vi "Main.vi"(8 "error":errorcluster) -> (0 "Error out":errorcluster)   [LabVIEW 2018, in "S1.lvclass"]
doc: "Use this template to build a simple state machine design pattern. Each state executes code and determines which state to transition to."
uses:
  S1.lvclass
  S1.lvclass/S1.ctl
  Controller/Public Controls/S1Config.ctl
  Controller/Public Controls/GlobalConfig.ctl
  Public Controls/Outputs.ctl
  Public Controls/ReportHeader.ctl
  Controller/Public Controls/TestInfo.ctl
  ce2ffe4b-55ea-4b97-aeef-069ef36f3054.vi
  18d9e863-2333-4af4-97b0-9e95cfa094dc.vi
  <vilib>/Utility/file.llb/Write Delimited Spreadsheet (string).vi
  Controller/GUI.lvclass
  IO/IO.lvclass
panel:
  out "Loop":i32
  # "S1 MAIN"
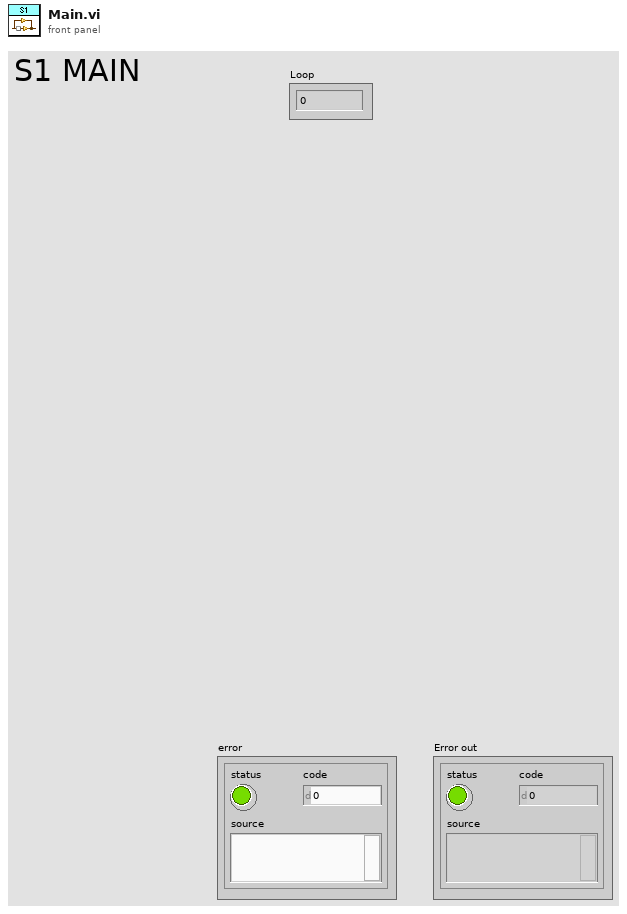
[diagram p1: front panel]
types:
  T1 = typedef "S1.lvclass/Outputs.ctl" = cluster{"LoP":bool, "HiP":bool, "Z1Vent":bool, "Z2Vent":bool, "Z3Vent":bool, "IsLidLock":bool}
  T2 = typedef "S1.lvclass/ReportHeader.ctl" = string
  T3 = typedef "GUI.lvclass/TestInfo.ctl" = cluster{"TestType":string, "SN":string}
  T4 = typedef "S1.lvclass/State.ctl" = enum16{"Initialize", "SetConfig", "AckAlarm", "Alarm", "Idle", "LockLid", "LowPressure", "HighPressure", "Vent", "Abort", "Start", "CreateReports", "WriteToReport", "WritePressure", "Error", "Exit"}
  T5 = typedef "GUI.lvclass/GlobalConfig.ctl" = cluster{"Report Folder Path":path, "PT1_MIN":dbl, "PT1_MAX":dbl, "VENT_PMAX":dbl, "LOP_TARGET":dbl, "LOP_RAMP":dbl, "LOP_LEAK_MAX":dbl, "HIP_TARGET":dbl, "HIP_RAMP":dbl, "HIP_MIN":dbl, "HIP_MAX":dbl, "BLEED_TIME":dbl, "LOP_MAX":dbl, "LOP_MIN":dbl, "PT131Com":refnum<visa-resource-name>, "PT231Com":refnum<visa-resource-name>, "PT331Com":refnum<visa-resource-name>, "PT431Com":refnum<visa-resource-name>, "PT531Com":refnum<visa-resource-name>, "PT631Com":refnum<visa-resource-name>}
  T6 = typedef "GUI.lvclass/S1Config.ctl" = cluster{"S1Z3_VENT_PMAX":dbl, "MSLOP_TIMER":dbl, "S1Z3_LOP_LEAK_MAX":dbl, "MSHIP_TIMER":dbl, "TJLOP_TIMER":dbl, "TJHIP_TIMER":dbl, "TJ_PTEST_MAX":dbl, "TJHIP_STABLE_WAIT":dbl, "TJHIP_STABLE_CLOSE":dbl}
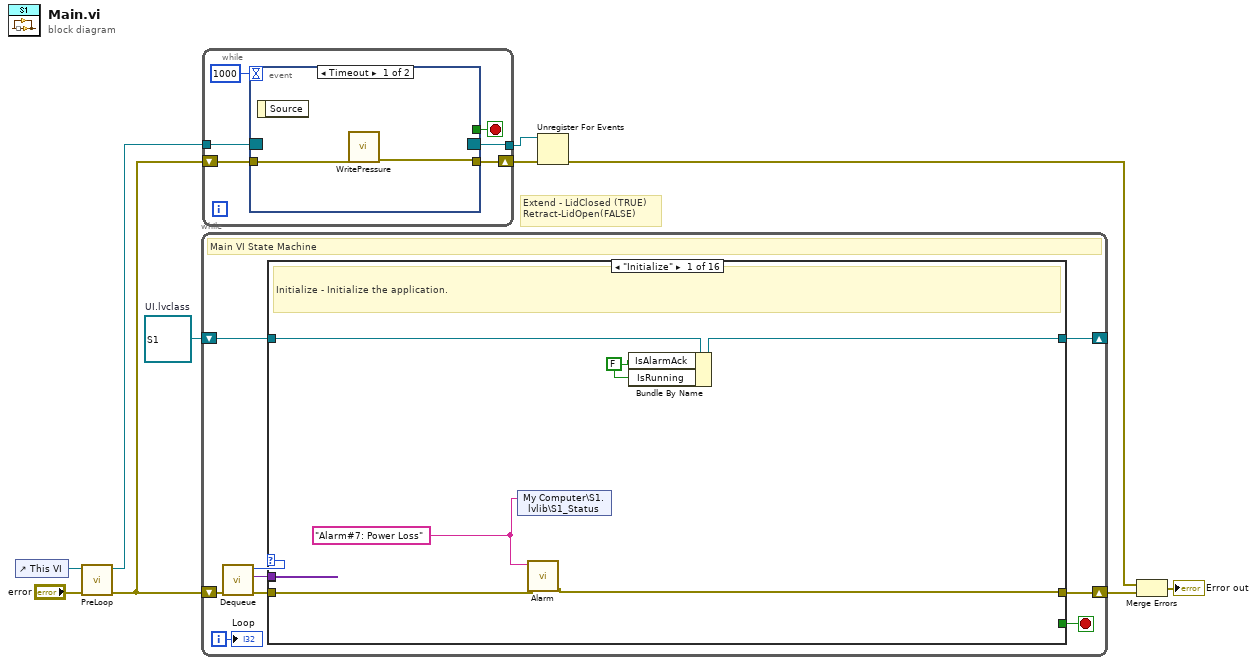
[diagram p0: block diagram]
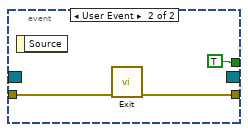
[diagram p2: hidden frame]
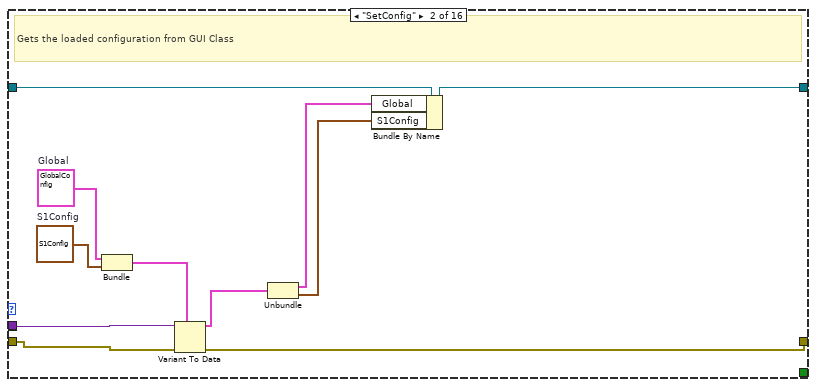
[diagram p3: hidden frame]
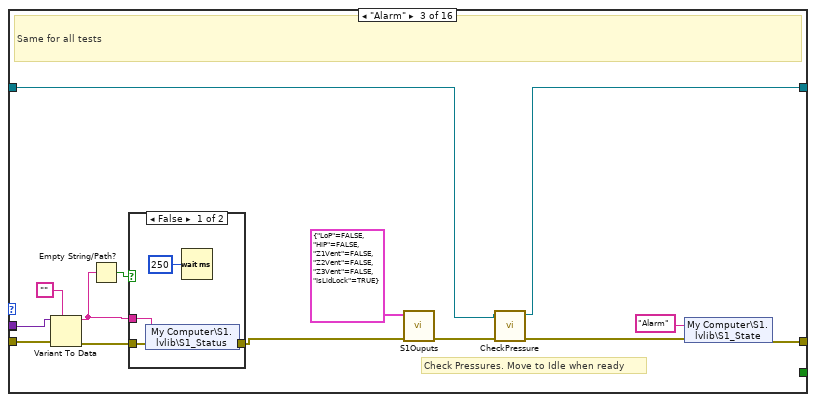
[diagram p4: hidden frame]
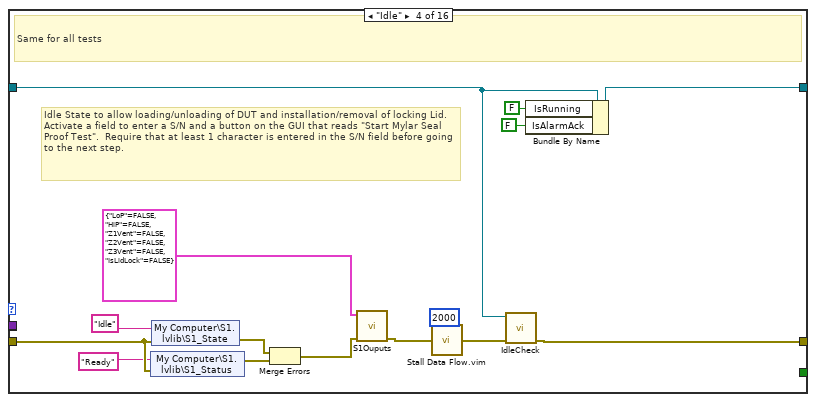
[diagram p6: hidden frame]
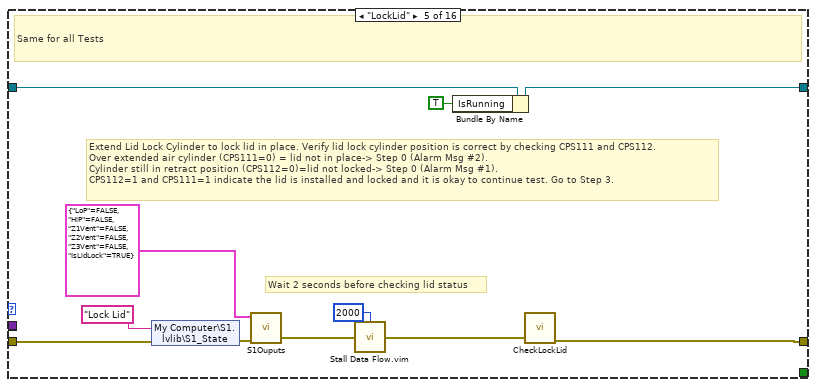
[diagram p7: hidden frame]
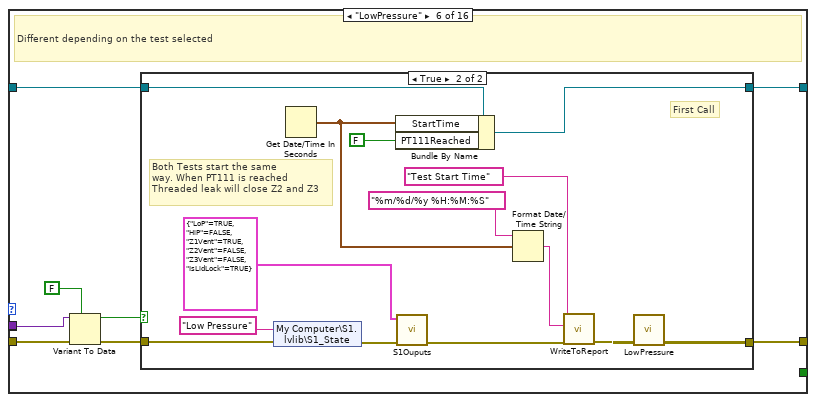
[diagram p8: hidden frame]
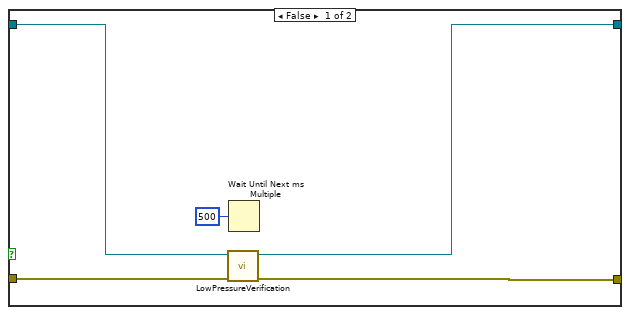
[diagram p9: hidden frame]
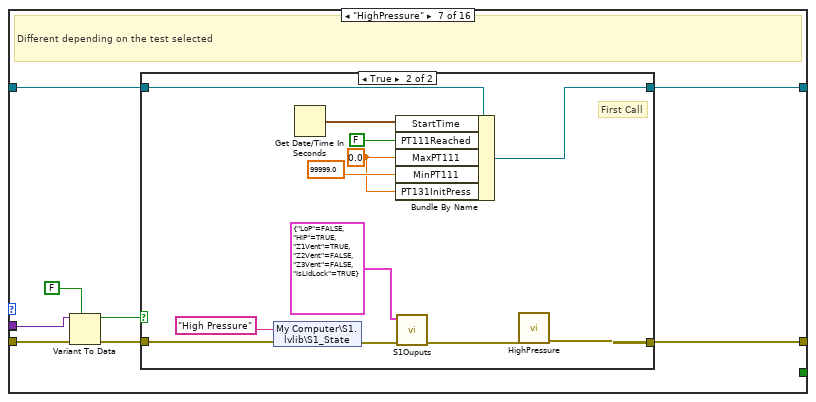
[diagram p10: hidden frame]
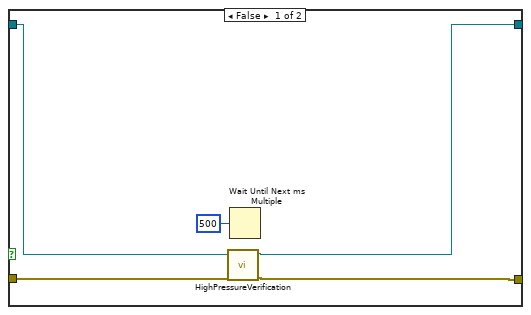
[diagram p11: hidden frame]
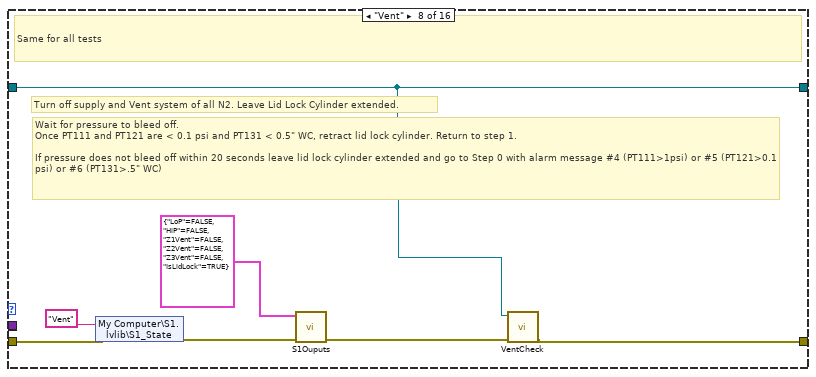
[diagram p12: hidden frame]
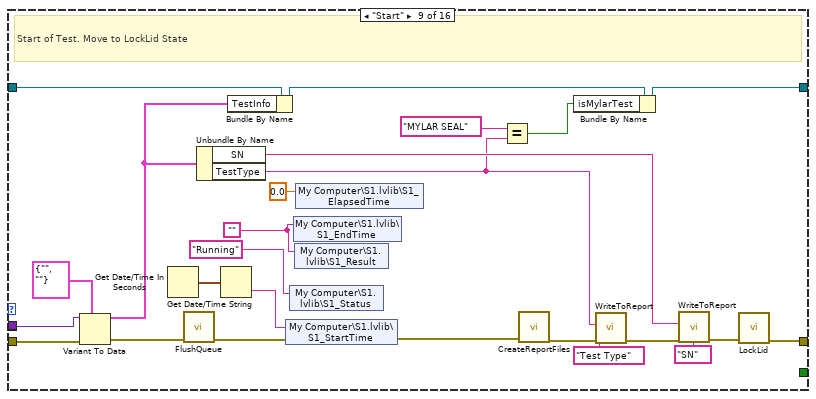
[diagram p13: hidden frame]
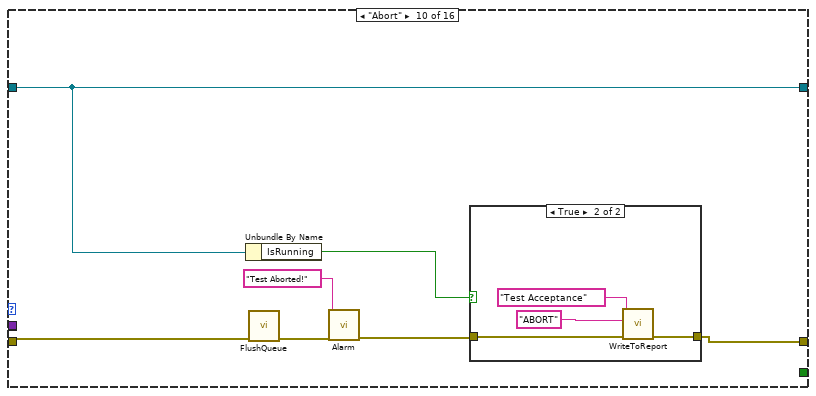
[diagram p14: hidden frame]
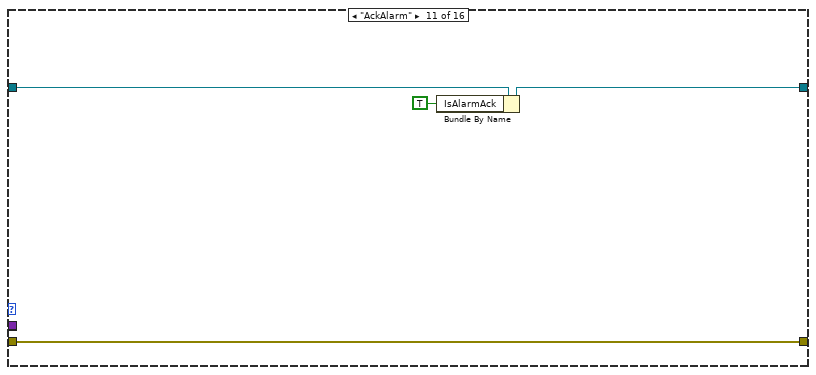
[diagram p16: hidden frame]
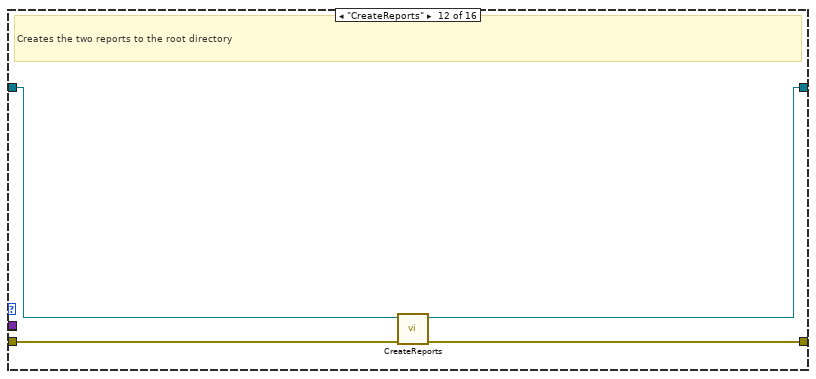
[diagram p17: hidden frame]
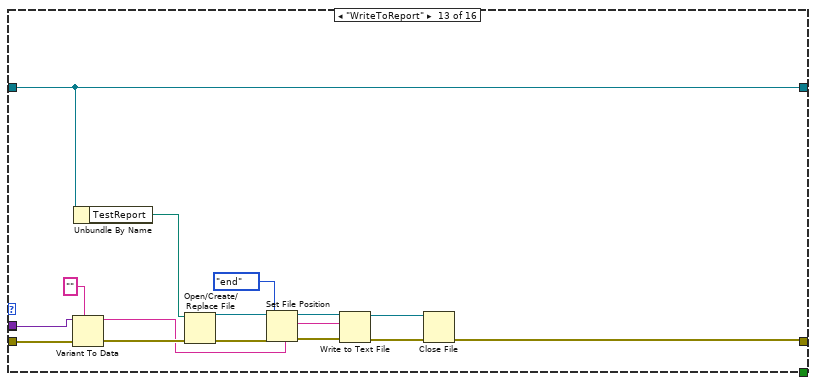
[diagram p18: hidden frame]
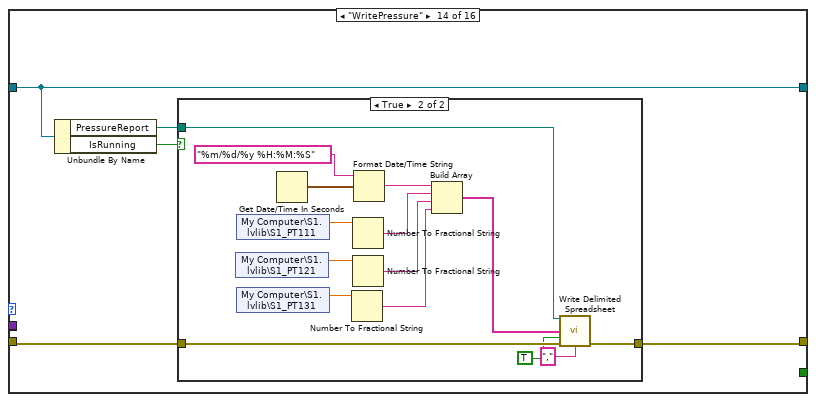
[diagram p19: hidden frame]
diagram:
  w10 = refnum<class "S1.lvclass"> refnum  # UI.lvclass
  # "Extend - LidClosed (TRUE)\nRetract-LidOpen(FALSE)"
  n1 = control-ref of="This VI"() -> (w7:refnum<vi>)
  n2 = call "PreLoop.vi"("error in"="error", "VI Ref"=w7) -> ("error out"=w6:errorcluster, "Event Registration Refnum"=w8:refnum<event-registration>)  [unwired: 8 in]
  n3 = while {
    shift-right: [w19] -> w3
    shift-left: w6 -> [w15]
    shift-right: [w16] -> _
    shift-left: w10 -> [w17]
    i -> [w11]
    stop <- w18 stop-if-true
    # "Main VI State Machine"
    n4 = call "Dequeue.vi"("error in"=w15) -> ("error out"=w14:errorcluster, "Data"=w12:variant, "State"=w13:T4)  [unwired: 8 in]
    n5 = case shown="\"Initialize\"" w13 {
      tunnel: [_ _ _ _ _ _ _ _ _ _ _ _ _ _ w224 _] -> w18
      tunnel: w14 -> [w23 w35 w43 w68 w80 w88 w115 w140 w161 w166 w181 w184 w198 w204 w222 w230]
      tunnel: [w22 w26 w44 w60 w76 w89 w116 w136 w150 w170 w181 w183 w191 w203 w222 w226] -> w19
      tunnel: w17 -> [w25 w36 w47 w56 w81 w83 w110 w134 w165 w169 w180 w185 w197 w205 w223 w233]
      tunnel: [w24 w30 w46 w63 w73 w82 w109 w134 w144 w169 w179 w182 w197 w205 w223 w233] -> w16
      tunnel: w12 -> [_ w34 w42 _ _ w87 w114 _ w159 _ _ _ w199 _ _ w229]
      tunnel: w12 -> [_ _ _ _ _ _ _ _ _ _ _ _ _ _ _ _]
      frame "Initialize" {
        w20 = FALSE ("IsAlarmAck")
        w21 = "Alarm#7: Power Loss" ("Status")
        # "Initialize - Initialize the application."
        n6 = shared-variable "My Computer\\S1.lvlib\\S1_Status"(w21) -> ()  [unwired: 1 in, 1 out]
        n7 = call "Alarm.vi"("error in"=w23, "Alarm"=w21) -> ("error out"=w22:errorcluster)  [unwired: 9 in]
        n8 = Bundle By Name(cluster=w25, "IsAlarmAck"=w20, "IsRunning"=w20) -> (w24:refnum<class "S1.lvclass">)
      }
      frame "SetConfig" {
        w33 = T5 {"Report Folder Path"=path "", "PT1_MIN"=0.0, "PT1_MAX"=0.0, "VENT_PMAX"=0.0, "LOP_TARGET"=0.0, "LOP_RAMP"=0.0, "LOP_LEAK_MAX"=0.0, "HIP_TARGET"=0.0, "HIP_RAMP"=0.0, "HIP_MIN"=0.0, "HIP_MAX"=0.0, "BLEED_TIME"=0.0, "LOP_MAX"=0.0, "LOP_MIN"=0.0, "PT131Com"="COM5", "PT231Com"="COM6", "PT331Com"="COM7", "PT431Com"="COM8", "PT531Com"="COM9", "PT631Com"="COM10"}  # Global
        w32 = T6 {"S1Z3_VENT_PMAX"=0.0, "MSLOP_TIMER"=0.0, "S1Z3_LOP_LEAK_MAX"=0.0, "MSHIP_TIMER"=0.0, "TJLOP_TIMER"=0.0, "TJHIP_TIMER"=0.0, "TJ_PTEST_MAX"=0.0, "TJHIP_STABLE_WAIT"=0.0, "TJHIP_STABLE_CLOSE"=0.0}  # S1Config
        # "Gets the loaded configuration from GUI Class"
        n9 = Bundle("Global"=w33, "S1Config"=w32) -> (w31:cluster{"Global":T5, "S1Config":T6})  [unwired: 1 in]
        n10 = Variant To Data(error in=w35, type=w31, Variant=w34) -> (data=w29:cluster{"Global":T5, "S1Config":T6}, error out=w26:errorcluster)
        n11 = Unbundle(w29) -> ("Global"=w28:T5, "S1Config"=w27:T6)
        n12 = Bundle By Name(cluster=w36, "Global"=w28, "S1Config"=w27) -> (w30:refnum<class "S1.lvclass">)
      }
      frame "Alarm" {
        # "Check Pressures. Move to Idle when ready"
        # "Same for all tests"
        n13 = Variant To Data(error in=w43, type="", Variant=w42) -> (data=w39:string, error out=w38:errorcluster)
        n14 = Empty String/Path?(string/path=w39) -> (empty?=w40:bool)
        n15 = case shown="False" w40 {
          tunnel: w39 -> [w54 _]
          tunnel: w38 -> [w53 w55]
          tunnel: [w52 w55] -> w37
          frame False {
            n16 = shared-variable "My Computer\\S1.lvlib\\S1_Status"(w54, error in=w53) -> (error out=w52:errorcluster)
            n17 = Wait (ms)(milliseconds to wait=u32 250) -> ()  [unwired: 1 out]
          }
          frame True {
          }
        }
        n18 = call "S1Ouputs.vi"("error in"=w37, "SIOutputs"=T1 {"LoP"=FALSE, "HiP"=FALSE, "Z1Vent"=FALSE, "Z2Vent"=FALSE, "Z3Vent"=FALSE, "IsLidLock"=TRUE}) -> ("error out"=w48:errorcluster)  [unwired: 9 in]
        n19 = call "CheckPressure.vi"("error in (no error)"=w48, "UI.lvclass"=w47) -> ("error out"=w45:errorcluster, "UI.lvclass"=w46:refnum<class "S1.lvclass">)  [unwired: 8 in]
        n20 = shared-variable "My Computer\\S1.lvlib\\S1_State"("Alarm" ("S1Status"), error in=w45) -> (error out=w44:errorcluster)
      }
      frame "Idle" {
        # "Idle State to allow loading/unloading of DUT and installation/removal of locking Lid.  Activate a field to enter a S/N and a button on the GUI that reads \"Start Mylar Seal Proof Test\".  Require that at least 1 character is entered in the S/N field before going to the next step."
        # "Same for all tests"
        n21 = shared-variable "My Computer\\S1.lvlib\\S1_Status"("Ready" ("Status"), error in=w68) -> (error out=w66:errorcluster)
        n22 = shared-variable "My Computer\\S1.lvlib\\S1_State"("Idle" ("S1Status"), error in=w68) -> (error out=w67:errorcluster)
        n23 = Merge Errors(w67, w66) -> (w65:errorcluster)
        n24 = call "S1Ouputs.vi"("error in"=w65, "SIOutputs"=T1 {"LoP"=FALSE, "HiP"=FALSE, "Z1Vent"=FALSE, "Z2Vent"=FALSE, "Z3Vent"=FALSE, "IsLidLock"=FALSE}) -> ("error out"=w61:errorcluster)  [unwired: 9 in]
        n25 = call "Stall Data Flow.vim"("value in"=w61, "milliseconds to wait"=u32 2000) -> ("value out"=w58:errorcluster)  [unwired: 1 out]
        n26 = call "IdleCheck.vi"("error in (no error)"=w58, "S1.lvclass"=w56) -> ("error out"=w60:errorcluster)  [unwired: 9 in]
        n27 = Bundle By Name(cluster=w56, "IsRunning"=FALSE, "IsAlarmAck"=FALSE) -> (w63:refnum<class "S1.lvclass">)
      }
      frame "LockLid" {
        # "Wait 2 seconds before checking lid status"
        # "Extend Lid Lock Cylinder to lock lid in place. Verify lid lock cylinder position is correct by checking CPS111 and CPS112. \nOver extended air cylinder (CPS111=0) = lid not in place-> Step 0 (Alarm Msg #2). \nCylinder still in retract position (CPS112=0)=lid not locked-> Step 0 (Alarm Msg #1). \nCPS112=1 and CPS111=1 indicate the lid is installed and locked and it is okay to continue test. Go to Step 3."
        # "Same for all Tests"
        n28 = shared-variable "My Computer\\S1.lvlib\\S1_State"("Lock Lid" ("S1Status"), error in=w80) -> (error out=w78:errorcluster)
        n29 = call "S1Ouputs.vi"("error in"=w78, "SIOutputs"=T1 {"LoP"=FALSE, "HiP"=FALSE, "Z1Vent"=FALSE, "Z2Vent"=FALSE, "Z3Vent"=FALSE, "IsLidLock"=TRUE}) -> ("error out"=w75:errorcluster)  [unwired: 9 in]
        n30 = call "Stall Data Flow.vim"("value in"=w75, "milliseconds to wait"=u32 2000) -> ("value out"=w74:errorcluster)  [unwired: 1 out]
        n31 = Bundle By Name(cluster=w81, "IsRunning"=TRUE) -> (w73:refnum<class "S1.lvclass">)
        n32 = call "CheckLockLid.vi"("error in (no error)"=w74) -> ("error out"=w76:errorcluster)  [unwired: 10 in]
      }
      frame "LowPressure" {
        # "Different depending on the test selected"
        n33 = Variant To Data(error in=w88, type=FALSE, Variant=w87) -> (data=w84:bool, error out=w85:errorcluster)
        n34 = case shown="True" w84 {
          tunnel: [w93 w95] -> w89
          tunnel: w85 -> [w94 w106]
          tunnel: w83 -> [w92 w99]
          tunnel: [w91 w105] -> w82
          frame False {
            n35 = call "LowPressureVerification.vi"("error in"=w94, "S1 in"=w92) -> ("error out"=w93:errorcluster, "S1 out"=w91:refnum<class "S1.lvclass">)  [unwired: 8 in]
            n36 = Wait Until Next ms Multiple(millisecond multiple=u32 500) -> ()  [unwired: 1 out]
          }
          frame True {
            # "Both Tests start the same\nway. When PT111 is reached\nThreaded leak will close Z2 and Z3"
            # "First Call"
            n37 = shared-variable "My Computer\\S1.lvlib\\S1_State"("Low Pressure" ("S1Status"), error in=w106) -> (error out=w107:errorcluster)
            n38 = Get Date/Time In Seconds() -> (seconds since 1Jan1904=w102:timestamp)
            n39 = Bundle By Name(cluster=w99, "StartTime"=w102, "PT111Reached"=FALSE ("PT111ReachedPressure")) -> (w105:refnum<class "S1.lvclass">)
            n40 = call "S1Ouputs.vi"("error in"=w107, "SIOutputs"=T1 {"LoP"=TRUE, "HiP"=FALSE, "Z1Vent"=TRUE, "Z2Vent"=FALSE, "Z3Vent"=FALSE, "IsLidLock"=TRUE}) -> ("error out"=w97:errorcluster)  [unwired: 9 in]
            n41 = Format Date/Time String(time format string (%c)="%m/%d/%y %H:%M:%S", seconds (now)=w102) -> (date/time string=w101:string)  [unwired: 1 in]
            n42 = call "WriteToReport.vi"("error in"=w97, "Value"=w101, "Header"=T2 "Test Start Time") -> ("error out"=w96:errorcluster)  [unwired: 8 in]
            n43 = call "LowPressure.vi"("error in"=w96) -> ("error out"=w95:errorcluster)  [unwired: 10 in]
          }
        }
      }
      frame "HighPressure" {
        # "Different depending on the test selected"
        n44 = Variant To Data(error in=w115, type=FALSE, Variant=w114) -> (data=w111:bool, error out=w112:errorcluster)
        n45 = case shown="True" w111 {
          tunnel: [w118 w125] -> w116
          tunnel: w112 -> [w119 w131]
          tunnel: w110 -> [w121 w124]
          tunnel: [w120 w130] -> w109
          frame False {
            n46 = call "HighPressureVerification.vi"("error in"=w119, "S1 in"=w121) -> ("error out"=w118:errorcluster, "S1 out"=w120:refnum<class "S1.lvclass">)  [unwired: 8 in]
            n47 = Wait Until Next ms Multiple(millisecond multiple=u32 500) -> ()  [unwired: 1 out]
          }
          frame True {
            w122 = 0.0 ("MaxPT111")
            # "First Call"
            n48 = shared-variable "My Computer\\S1.lvlib\\S1_State"("High Pressure" ("S1Status"), error in=w131) -> (error out=w132:errorcluster)
            n49 = Get Date/Time In Seconds() -> (seconds since 1Jan1904=w129:timestamp)
            n50 = Bundle By Name(cluster=w124, "StartTime"=w129, "PT111Reached"=FALSE ("PT111ReachedPressure"), "MaxPT111"=w122, "MinPT111"=99999.0, "PT131InitPress"=w122) -> (w130:refnum<class "S1.lvclass">)
            n51 = call "S1Ouputs.vi"("error in"=w132, "SIOutputs"=T1 {"LoP"=FALSE, "HiP"=TRUE, "Z1Vent"=TRUE, "Z2Vent"=FALSE, "Z3Vent"=FALSE, "IsLidLock"=TRUE}) -> ("error out"=w128:errorcluster)  [unwired: 9 in]
            n52 = call "HighPressure.vi"("error in"=w128) -> ("error out"=w125:errorcluster)  [unwired: 10 in]
          }
        }
      }
      frame "Vent" {
        # "Wait for pressure to bleed off. \nOnce PT111 and PT121 are < 0.1 psi and PT131 < 0.5\" WC, retract lid lock cylinder. Return to step 1. \n\nIf pressure does not bleed off within 20 seconds leave lid lock cylinder extended and go to Step 0 with alarm message #4 (PT111>1psi) or #5 (PT121>0.1 psi) or #6 (PT131>.5\" WC)"
        # "Turn off supply and Vent system of all N2. Leave Lid Lock Cylinder extended."
        # "Same for all tests"
        n53 = shared-variable "My Computer\\S1.lvlib\\S1_State"("Vent" ("S1Status"), error in=w140) -> (error out=w138:errorcluster)
        n54 = call "S1Ouputs.vi"("error in"=w138, "SIOutputs"=T1 {"LoP"=FALSE, "HiP"=FALSE, "Z1Vent"=FALSE, "Z2Vent"=FALSE, "Z3Vent"=FALSE, "IsLidLock"=TRUE}) -> ("error out"=w135:errorcluster)  [unwired: 9 in]
        n55 = call "VentCheck.vi"("error in (no error)"=w135, "UI.lvclass"=w134) -> ("error out"=w136:errorcluster)  [unwired: 9 in]
      }
      frame "Start" {
        w147 = ""
        # "Start of Test. Move to LockLid State"
        n56 = Variant To Data(error in=w161, type=T3 {"TestType"="", "SN"=""} ("TestInfo"), Variant=w159) -> (data=w155:T3, error out=w142:errorcluster)
        n57 = Get Date/Time In Seconds() -> (seconds since 1Jan1904=w164:timestamp)
        n58 = call "FlushQueue.vi"("error in"=w142) -> ("error out"=w141:errorcluster)  [unwired: 10 in]
        n59 = Unbundle By Name(w155) -> ("SN"=w153:string, "TestType"=w145:string)
        n60 = Get Date/Time String(seconds (now)=w164) -> (time string=w163:string)  [unwired: 2 in, 1 out]
        n61 = Bundle By Name(cluster=w165, "TestInfo"=w155) -> (w158:refnum<class "S1.lvclass">)
        n62 = shared-variable "My Computer\\S1.lvlib\\S1_StartTime"(w163, error in=w141) -> (error out=w149:errorcluster)
        n63 = shared-variable "My Computer\\S1.lvlib\\S1_Status"("Running" ("S1Status")) -> ()  [unwired: 1 in, 1 out]
        n64 = shared-variable "My Computer\\S1.lvlib\\S1_EndTime"(w147) -> ()  [unwired: 1 in, 1 out]
        n65 = shared-variable "My Computer\\S1.lvlib\\S1_Result"(w147) -> ()  [unwired: 1 in, 1 out]
        n66 = shared-variable "My Computer\\S1.lvlib\\S1_ElapsedTime"(0.0 ("ElapsedTime")) -> ()  [unwired: 1 in, 1 out]
        n67 = Equal?(x="MYLAR SEAL" ("TestInfo.TestType"), y=w145) -> (x = y?=w143:bool)
        n68 = call "CreateReportFiles.vi"("error in"=w149) -> ("error out"=w156:errorcluster)  [unwired: 10 in]
        n69 = Bundle By Name(cluster=w158, "isMylarTest"=w143) -> (w144:refnum<class "S1.lvclass">)
        n70 = call "WriteToReport.vi"("error in"=w156, "Value"=w145, "Header"="Test Type") -> ("error out"=w154:errorcluster)  [unwired: 8 in]
        n71 = call "WriteToReport.vi"("error in"=w154, "Value"=w153, "Header"="SN") -> ("error out"=w151:errorcluster)  [unwired: 8 in]
        n72 = call "LockLid.vi"("error in"=w151) -> ("error out"=w150:errorcluster)  [unwired: 10 in]
      }
      frame "Abort" {
        n73 = Unbundle By Name(w169) -> ("IsRunning"=w172:bool)
        n74 = call "FlushQueue.vi"("error in"=w166) -> ("error out"=w168:errorcluster)  [unwired: 10 in]
        n75 = call "Alarm.vi"("error in"=w168, "Alarm"="Test Aborted!" ("S1Status")) -> ("error out"=w171:errorcluster)  [unwired: 9 in]
        n76 = case shown="True" w172 {
          tunnel: w171 -> [w173 w177]
          tunnel: [w173 w176] -> w170
          frame False {
          }
          frame True {
            n77 = call "WriteToReport.vi"("error in"=w177, "Value"="ABORT", "Header"=T2 "Test Acceptance") -> ("error out"=w176:errorcluster)  [unwired: 8 in]
          }
        }
      }
      frame "AckAlarm" {
        n78 = Bundle By Name(cluster=w180, "IsAlarmAck"=TRUE) -> (w179:refnum<class "S1.lvclass">)
      }
      frame "CreateReports" {
        # "Creates the two reports to the root directory"
        n79 = call "CreateReports.vi"("error in (no error)"=w184, "S1 in"=w185) -> ("error out"=w183:errorcluster, "S1 out"=w182:refnum<class "S1.lvclass">)  [unwired: 8 in]
      }
      frame "WriteToReport" {
        n80 = Variant To Data(error in=w198, type="", Variant=w199) -> (data=w194:string, error out=w195:errorcluster)
        n81 = Unbundle By Name(w197) -> ("TestReport"=w196:path)
        n82 = Open/Create/Replace File(file path (use dialog)=w196, error in=w195) -> (refnum out=w187:refnum<file>, error out=w190:errorcluster)  [unwired: 4 in, 1 out]
        n83 = Set File Position(refnum=w187, from (0:start)=enum16{"start", "end", "current"}."end", error in=w190) -> (refnum out=w186:refnum<file>, error out=w188:errorcluster)  [unwired: 1 in]
        n84 = Write to Text File(file (use dialog)=w186, text=w194, error in=w188) -> (refnum out=w193:refnum<file>, error out=w192:errorcluster)  [unwired: 1 in, 1 out]
        n85 = Close File(refnum=w193, error in=w192) -> (error out=w191:errorcluster)  [unwired: 1 out]
      }
      frame "WritePressure" {
        n86 = Unbundle By Name(w205) -> ("PressureReport"=w201:path, "IsRunning"=w202:bool)
        n87 = case shown="True" w202 {
          tunnel: w204 -> [w206 w211]
          tunnel: [w206 w210] -> w203
          tunnel: w201 -> [_ w207]
          frame False {
          }
          frame True {
            n88 = shared-variable "My Computer\\S1.lvlib\\S1_PT121"() -> (w218:dbl)  [unwired: 1 in, 1 out]
            n89 = shared-variable "My Computer\\S1.lvlib\\S1_PT111"() -> (w219:dbl)  [unwired: 1 in, 1 out]
            n90 = shared-variable "My Computer\\S1.lvlib\\S1_PT131"() -> (w217:dbl)  [unwired: 1 in, 1 out]
            n91 = Get Date/Time In Seconds() -> (seconds since 1Jan1904=w221:timestamp)
            n92 = Number To Fractional String(number=w217) -> (F-format string=w213:string)  [unwired: 3 in]
            n93 = Number To Fractional String(number=w219) -> (F-format string=w215:string)  [unwired: 3 in]
            n94 = Number To Fractional String(number=w218) -> (F-format string=w214:string)  [unwired: 3 in]
            n95 = Format Date/Time String(time format string (%c)="%m/%d/%y %H:%M:%S", seconds (now)=w221) -> (date/time string=w216:string)  [unwired: 1 in]
            n96 = Build Array(w216, w215, w214, w213) -> (w212:string[])
            n97 = call-poly <vilib>:"Write Delimited Spreadsheet.vi"("file path (dialog if empty)"=w207, "1D data"=w212, "append to file? (new file:F)"=TRUE, "error in (no error)"=w211, "delimiter (\\t)"="," ("delimiter (\\t)")) -> ("error out"=w210:errorcluster)  [unwired: 9 in, 1 out]
          }
        }
      }
      frame "Exit" {
        w224 = TRUE  # Stop Loop
        # "Exit - Exit the application.\nSave / Close any files"
      }
      frame "Error" {
        n98 = Variant To Data(error in=w230, type=errorcluster {"status"=FALSE, "code"=0, "source"=""} ("error out"), Variant=w229) -> (data=w231:errorcluster, error out=w227:errorcluster)
        n99 = Unbundle By Name(w231) -> ("code"=w225:i32, "source"=w228:string)
        n100 = case shown="Default" w225 {
          tunnel: w228 -> [_ w235]
          tunnel: w227 -> [w234 w238]
          tunnel: [w234 w238] -> w226
          frame 1 {
            # "Error talking to other modules. \n\nIgnore. If testing by itself."
          }
          frame Default {
            n101 = Concatenate Strings("Error On Station 1 ", w235) -> (w237:string)
            n102 = One Button Dialog(message=w237) -> ()  [unwired: 1 in, 1 out]
          }
        }
      }
    }
    "Loop" <- w11
  }
  n103 = while {
    tunnel: w8 -> [w240]
    shift-right: [w242] -> w5
    shift-left: w6 -> [w244]
    tunnel: [w241] -> w4
    stop <- w243 stop-if-true
    n104 = event shown="[0] Timeout" {
      selector: w240 -> [_ _]
      dyn-events: [_ _] -> w241
      timeout: 1000 -> [_ _]
      tunnel: w244 -> [w246 w249]
      tunnel: [w245 w248] -> w242
      tunnel: [_ TRUE] -> w243
      event Timeout {
        n105 = event-data() -> ()  [unwired: 1 in, 1 out]
        n106 = call "WritePressure.vi"("error in"=w246) -> ("error out"=w245:errorcluster)  [unwired: 10 in]
      }
      event User Event {
        n107 = event-data() -> ()  [unwired: 1 in, 1 out]
        n108 = call "Exit.vi"("error in"=w249) -> ("error out"=w248:errorcluster)  [unwired: 10 in]
      }
    }
  }
  n109 = Unregister For Events(event registration refnum=w4, error in=w5) -> (error out=w2:errorcluster)
  n110 = Merge Errors(w2, w3) -> (→"Error out":errorcluster)
